vi "Field Delete.vi"(8 "error in (no error)":errorcluster, 10 "Field":T2={"ixField"=0, "iSequenceOrder"=0, "sxFieldId"="", "sxSequenceId"="", "sDisplayName"="", "sValue"="", "sUnits"="", "nDataType"=enum."timestamp", "nNextItem"=enum."Reset", "fSystem"=FALSE, "fSystemValue"=FALSE, "fRequired"=FALSE, "fSetAtTest"=FALSE, "fTestField"=FALSE, "fDeleted"=FALSE, "fIndexed"=FALSE, "fFreeList"=FALSE}, 11 "Connection Refnum":T1) -> (0 "error out":errorcluster, 3 "Connection Refnum":T1)   [LabVIEW 2011]
uses:
  Field Record.ctl
  Field DataTypes.ctl
  Field NextItem.ctl
  Summitek EXT/ODBC/SQL Controls/Connection Refnum.ctl
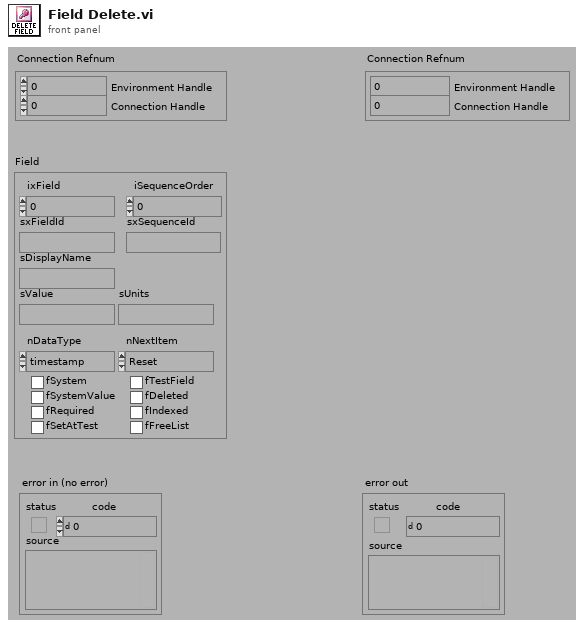
[diagram p1: front panel]
types:
  T1 = typedef "Connection Refnum.ctl" = cluster{"Environment Handle":i32, "Connection Handle":i32}
  T2 = typedef "Field Record.ctl" = cluster{"ixField":i32, "iSequenceOrder":i32, "sxFieldId":string, "sxSequenceId":string, "sDisplayName":string, "sValue":string, "sUnits":string, "nDataType":T3, "nNextItem":T4, "fSystem":bool, "fSystemValue":bool, "fRequired":bool, "fSetAtTest":bool, "fTestField":bool, "fDeleted":bool, "fIndexed":bool, "fFreeList":bool}
  T3 = typedef "Field DataTypes.ctl" = enum32{"text", "numeric", "list", "timestamp", "boolean"}
  T4 = typedef "Field NextItem.ctl" = enum32{"Reset", "Retain", "Auto-Increment"}
  T5 = typedef "Statement Refnum.ctl" = cluster{"Statement Handle":i32, "Parameter Number":u16}
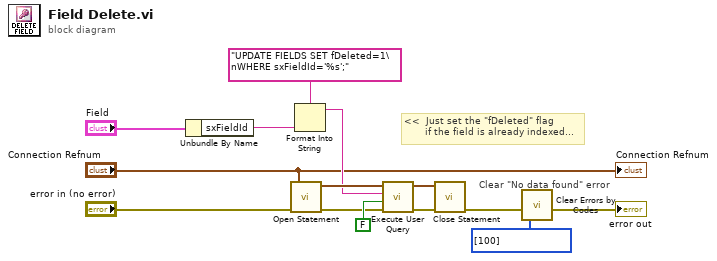
[diagram p0: block diagram]
diagram:
  # "<<  Just set the \"fDeleted\" flag\n       if the field is already indexed..."
  # "Clear \"No data found\" error"
  n1 = Unbundle By Name("Field") -> ("sxFieldId"=w10:string)
  n2 = call "Open Statement.vi"("error in (no error)"="error in (no error)", "Connection Refnum"="Connection Refnum") -> ("error out"=w9:errorcluster, "Statement Refnum"=w8:T5)  [unwired: 4 out]
  n3 = Format Into String(format string="UPDATE FIELDS SET fDeleted=1\nWHERE sxFieldId='%s';" ("User Query"), w10) -> (resulting string=w7:string)  [unwired: 2 in, 1 out]
  n4 = call "Execute User Query.vi"("error in (no error)"=w9, "Return Data? (f)"=FALSE, "User Query"=w7, "Statement Refnum"=w8) -> ("error out"=w11:errorcluster, "Statement Refnum"=w12:T5)  [unwired: 2 out]
  n5 = call "Close Statement.vi"("error in (no error)"=w11, "Statement Refnum"=w12) -> ("error out"=w5:errorcluster)  [unwired: 5 out]
  n6 = call "Clear Errors by Codes.vi"("Error Codes\nto Clear (Empty)"=i32[] [100] ("Error Codes\nto Clear (Empty)"), "error in (no error)"=w5) -> ("error out"=→"error out":errorcluster)  [unwired: 5 out]
  "Connection Refnum" <- "Connection Refnum"
